vi "TIO Data Stream Parse pstream Info.vi"(8 "pstreams in":T2(array[cluster]), 11 "pstream info raw":string="\u0000\u0000\u0001\u0000\u0001\u0000\u0000\u0000\u0000\u0000\u0000\u0000ÿÿÿÿ\u0000\u0000\u0003\u0000Bgmr\tx,y,z\tVector magnetic field\tnT") -> (0 "pstreams out":T2(array[cluster]))   [LabVIEW 2012]
panel:
  out "pstream info":T1
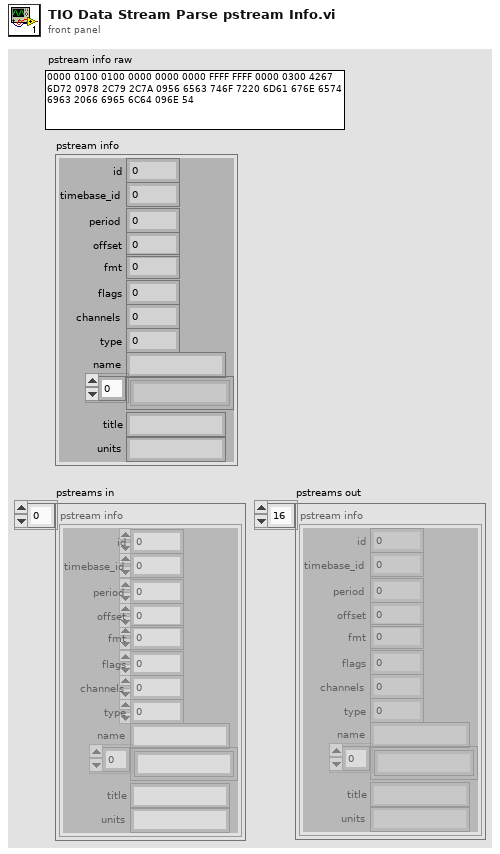
[diagram p1: front panel]
types:
  T1 = cluster{"id":u16, "timebase_id":u16, "period":u32, "offset":u32, "fmt":i32, "flags":u16, "channels":u16, "type":u8, "name":string, string[], "title":string, "units":string}
  T2 = cluster{"id":u16, "timebase_id":u16, "period":u32, "offset":u32, "fmt":i32, "flags":u16, "channels":u16, "type":u8, "name":string, string[], "title":string, "units":string}[]
  T3 = enum16{"big-endian, network order", "native, host order", "little-endian"}
  T4 = cluster{"u16":u16, "u16":u16, "u32":u32, "u32":u32, "i32":i32, "u16":u16, "u16":u16, "u8":u8}
  T5 = cluster{"u16":u16, "u16":u16, "u32":u32, "u32":u32, "i32":i32, "u16":u16, "u16":u16, "u8":u8, string, string[], string, string}
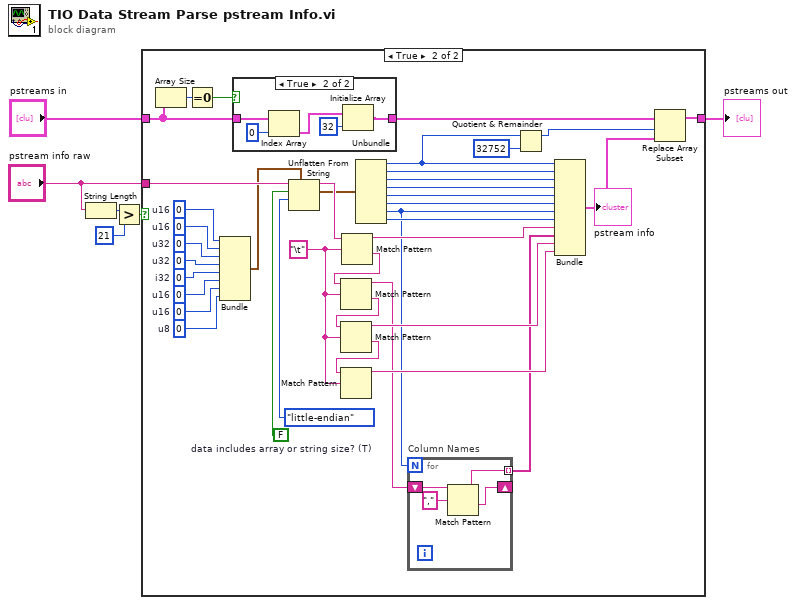
[diagram p0: block diagram]
diagram:
  n1 = String Length(string="pstream info raw") -> (length=w5:i32)
  n2 = Greater?(x=w5, y=21) -> (0:w4:bool)
  n3 = case shown="True" w4 {
    tunnel: "pstream info raw" -> [_ w46]
    tunnel: "pstreams in" -> [w7 w14]
    tunnel: [w7 w12] -> w1
    frame False {
    }
    frame True {
      w24 = "\t" ("regular expression")
      w38 = u8 0  # u8
      w21 = u16 0  # u16
      w39 = u16 0  # u16
      w40 = 0  # i32
      w41 = u32 0  # u32
      w42 = u32 0  # u32
      w43 = u16 0  # u16
      w17 = u16 0  # u16
      w45 = FALSE  # data includes array or string size? (T)
      n4 = Array Size(array=w14) -> (size(s)=w16:i32)
      n5 = Equal To 0?(x=w16) -> (x = 0?=w15:bool)
      n6 = Bundle("u16"=w17, "u16"=w43, "u32"=w42, "u32"=w41, "i32"=w40, "u16"=w39, "u16"=w21, "u8"=w38) -> (w37:T4)  [unwired: 1 in]
      n7 = case shown="True" w15 {
        tunnel: [w47 w52] -> w13
        tunnel: w14 -> [w47 w50]
        frame False {
        }
        frame True {
          n8 = Index Array(array=w50, index=0) -> (element=w48:T1)
          n9 = Initialize Array(w48, 32 ("dimension size")) -> (w52:T2)
        }
      }
      n10 = Unflatten From String(type=w37, binary string=w46, data includes array or string size? (T)=w45, byte order (0:big-endian, network order)=T3."little-endian") -> (rest of the binary string=w36:string, value=w22:T4)  [unwired: 1 in, 1 out]
      n11 = Match Pattern(string=w36, regular expression=w24) -> (before substring=w29:string, after substring=w28:string)  [unwired: 1 in, 2 out]
      n12 = Match Pattern(string=w28, regular expression=w24) -> (before substring=w20:string, after substring=w27:string)  [unwired: 1 in, 2 out]
      n13 = Match Pattern(string=w27, regular expression=w24) -> (before substring=w26:string, after substring=w25:string)  [unwired: 1 in, 2 out]
      n14 = Match Pattern(string=w25, regular expression=w24) -> (before substring=w23:string)  [unwired: 1 in, 3 out]
      n15 = Unbundle(w22) -> ("u16"=w10:u16, "u16"=w35:u16, "u32"=w34:u32, "u32"=w33:u32, "i32"=w32:i32, "u16"=w31:u16, "u16"=w18:u16, "u8"=w30:u8)
      n16 = for "Column Names" {
        N: w18 -> [_]
        shift-right: [w54] -> _
        shift-left: w20 -> [w56]
        tunnel: [w53] -> w19 mode=indexing
        n17 = Match Pattern(string=w56, regular expression=",") -> (before substring=w53:string, after substring=w54:string)  [unwired: 1 in, 2 out]
      }
      n18 = Quotient & Remainder(x=w10, y=u16 32752) -> (x-y*floor(x/y)=w8:u16)  [unwired: 1 out]
      n19 = Bundle("u16"=w10, "u16"=w35, "u32"=w34, "u32"=w33, "i32"=w32, "u16"=w31, "u16"=w18, "u8"=w30, w29, w19, w26, w23) -> (w11:T5)  [unwired: 1 in]
      "pstream info" <- w11
      n20 = Replace Array Subset(array=w13, new element=w11, index=w8) -> (w12:T2)
    }
  }
  "pstreams out" <- w1
